vi "Teleop.vi"(10 "Match Info":T1={"Autonomous Elapsed Seconds"=0.0, "TeleOp Elapsed Seconds"=0.0, "Disabled Elapsed Seconds"=0.0, "Visited Autonomous"=FALSE, "Visited TeleOp"=FALSE, "Visited Disabled"=FALSE, "Autonomous Settings"={"Autonomous Style"=enum."Independent", "VI Refnum"=refnum}}, 11 "Call Context":T2) -> ()   [LabVIEW 2013]
doc: "This VI is called for each TeleOp packet received from the DS where the robot is not disabled. It is often used to read from the joysticks and update I/O or to update setpoints for timed control loops. It should complete and return within 20 milliseconds or it may miss DS packets."
uses:
  <vilib>/Rock Robotics/WPI/DriverStation/WPI_DriverStationDerivedRobotMode.ctl
  <vilib>/Rock Robotics/WPI/DriverStation/WPI_DriverStationMatch Info.ctl
  <vilib>/Rock Robotics/WPI/Solenoid/WPI_SolenoidValue.ctl
  <vilib>/Rock Robotics/WPI/Relay/WPI_RelayValue.ctl
  Robot Global Data.vi
  <vilib>/Rock Robotics/WPI/Joystick/WPI_JoystickGetSetRefNum.vi
  <vilib>/Rock Robotics/WPI/Solenoid/WPI_SolenoidSetEnum.vi
panel:
  in  "StatusOfFiringMechanism":enum16{"Retracting", "Extending", "Off", ""}(ring)=enum."Off"
  in  "PID Distance":dbl
  in  "Run PID":bool
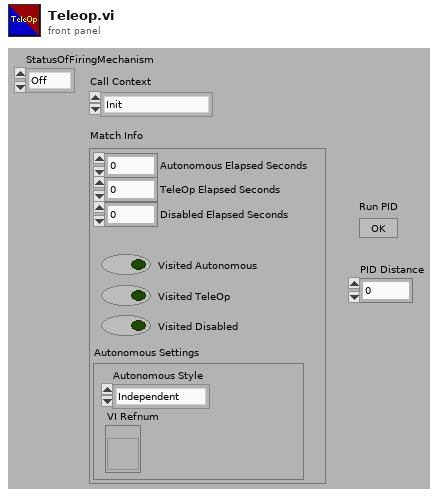
[diagram p1: front panel]
types:
  T1 = typedef "WPI_DriverStationMatch Info.ctl" = cluster{"Autonomous Elapsed Seconds":dbl, "TeleOp Elapsed Seconds":dbl, "Disabled Elapsed Seconds":dbl, "Visited Autonomous":bool, "Visited TeleOp":bool, "Visited Disabled":bool, "Autonomous Settings":cluster{"Autonomous Style":enum16{"Iterative", "Independent"}, "VI Refnum":refnum<vi>}}
  T2 = typedef "WPI_DriverStationDerivedRobotMode.ctl" = enum16{"Init", "Execute", "Stop"}
  T3 = typedef "WPI_RelayDevRef.ctl" = cluster{"DevStatus":errorcluster, "Relay Channel":T4, "Digital Module":T5, "Relay Direction":T6}
  T4 = typedef "FPGA_DIORelayChannel.ctl" = enum8{"Relay 1", "Relay 2", "Relay 3", "Relay 4", "Relay 5", "Relay 6", "Relay 7", "Relay 8", "Invalid"}
  T5 = typedef "FPGA_TypedefDigitalModule.ctl" = enum16{"Digital Module 1", "Digital Module 2"}
  T6 = typedef "WPI_RelayDirection.ctl" = enum16{"Both directions", "Forward only", "Reverse only"}
  T7 = typedef "WPI_SolenoidDevRef.ctl" = cluster{"DevStatus":errorcluster, "Solenoid Module":T8, "Forward Solenoid Channel":T9, "Reverse Solenoid Channel":T9}
  T8 = typedef "FPGA_TypedefSolenoidModule.ctl" = enum16{"Solenoid Module 1", "Solenoid Module 2"}
  T9 = typedef "WPI_SolenoidChannel.ctl" = enum8{"Solenoid 1", "Solenoid 2", "Solenoid 3", "Solenoid 4", "Solenoid 5", "Solenoid 6", "Solenoid 7", "Solenoid 8", "Invalid"}
  T10 = typedef "WPI_RelayValue.ctl" = enum16{"Off", "On", "Forward", "Reverse"}
  T11 = typedef "WPI_SolenoidValue.ctl" = enum16{"Off", "On", "Forward", "Reverse"}
  T12 = typedef "WPI_MotorControlDeviceRef.ctl" = cluster{"DeviceStatus":errorcluster, "Type":enum16{"PWM", "CAN"}, "PWM":cluster{"Digital Module":T5, "PWM Channel":T13, "DeadBand":T14}, "CAN":cluster{"Device Number":u8, "Control Mode":T15, "Semaphore":T16, "Max Vout":dbl}, "Invert":bool, "TransformRef":T17, "InvTransformRef":T17}
  T13 = typedef "FPGA_DIOPWMChannel.ctl" = enum8{"PWM 1", "PWM 2", "PWM 3", "PWM 4", "PWM 5", "PWM 6", "PWM 7", "PWM 8", "PWM 9", "PWM 10", "Invalid"}
  T14 = typedef "WPI_PWMDeadband.ctl" = cluster{"Name":string, "maxPositivePwm":i32, "minPositivePwm":i32, "centerPwm":i32, "maxNegativePwm":i32, "minNegativePwm":i32, "angularRange":u16}
  T15 = typedef "WPI_CANJaguar_ControlMode.ctl" = enum8{"Percent VBus", "Current", "Speed", "Position", "Voltage"}
  T16 = typedef "Semaphore RefNum" = refnum<k1>
  T17 = typedef "WPI_PWMTransform_ConPane.ctl" = refnum<vi>
  T18 = typedef "WPI_RobotDriveDevRef.ctl" = cluster{"DevStatus":errorcluster, "Motors[]":T12[], "Square Inputs":bool, "Max Output":dbl, "Isochronous":bool}
  T19 = typedef "WPI_JoystickDevRef.ctl" = cluster{"Device":T20}
  T20 = typedef "WPI_JoystickDeviceEnum.ctl" = enum16{"USB 1", "USB 2", "USB 3", "USB 4", "Kinect 1", "Kinect 2"}
  T21 = typedef "WPI_JoystickButtonState.ctl" = cluster{"Button 1":bool, "Button 2":bool, "Button 3":bool, "Button 4":bool, "Button 5":bool, "Button 6":bool, "Button 7":bool, "Button 8":bool, "Button 9":bool, "Button 10":bool, "Button 11":bool, "Button 12":bool}
  T22 = cluster{"axis 1 (x)":dbl, "axis 2 (y)":dbl, "axis 3 (throttle)":dbl, "axis 4":dbl, "axis 5":dbl, "axis 6":dbl}
  T23 = typedef "WPI_DigitalInputDevRef.ctl" = cluster{"DevStatus":errorcluster, "DIO Channel":T24, "Digital Module":T5}
  T24 = typedef "FPGA_DIOChannel.ctl" = enum8{"DIO 1", "DIO 2", "DIO 3", "DIO 4", "DIO 5", "DIO 6", "DIO 7", "DIO 8", "DIO 9", "DIO 10", "DIO 11", "DIO 12", "DIO 13", "DIO 14", "Invalid"}
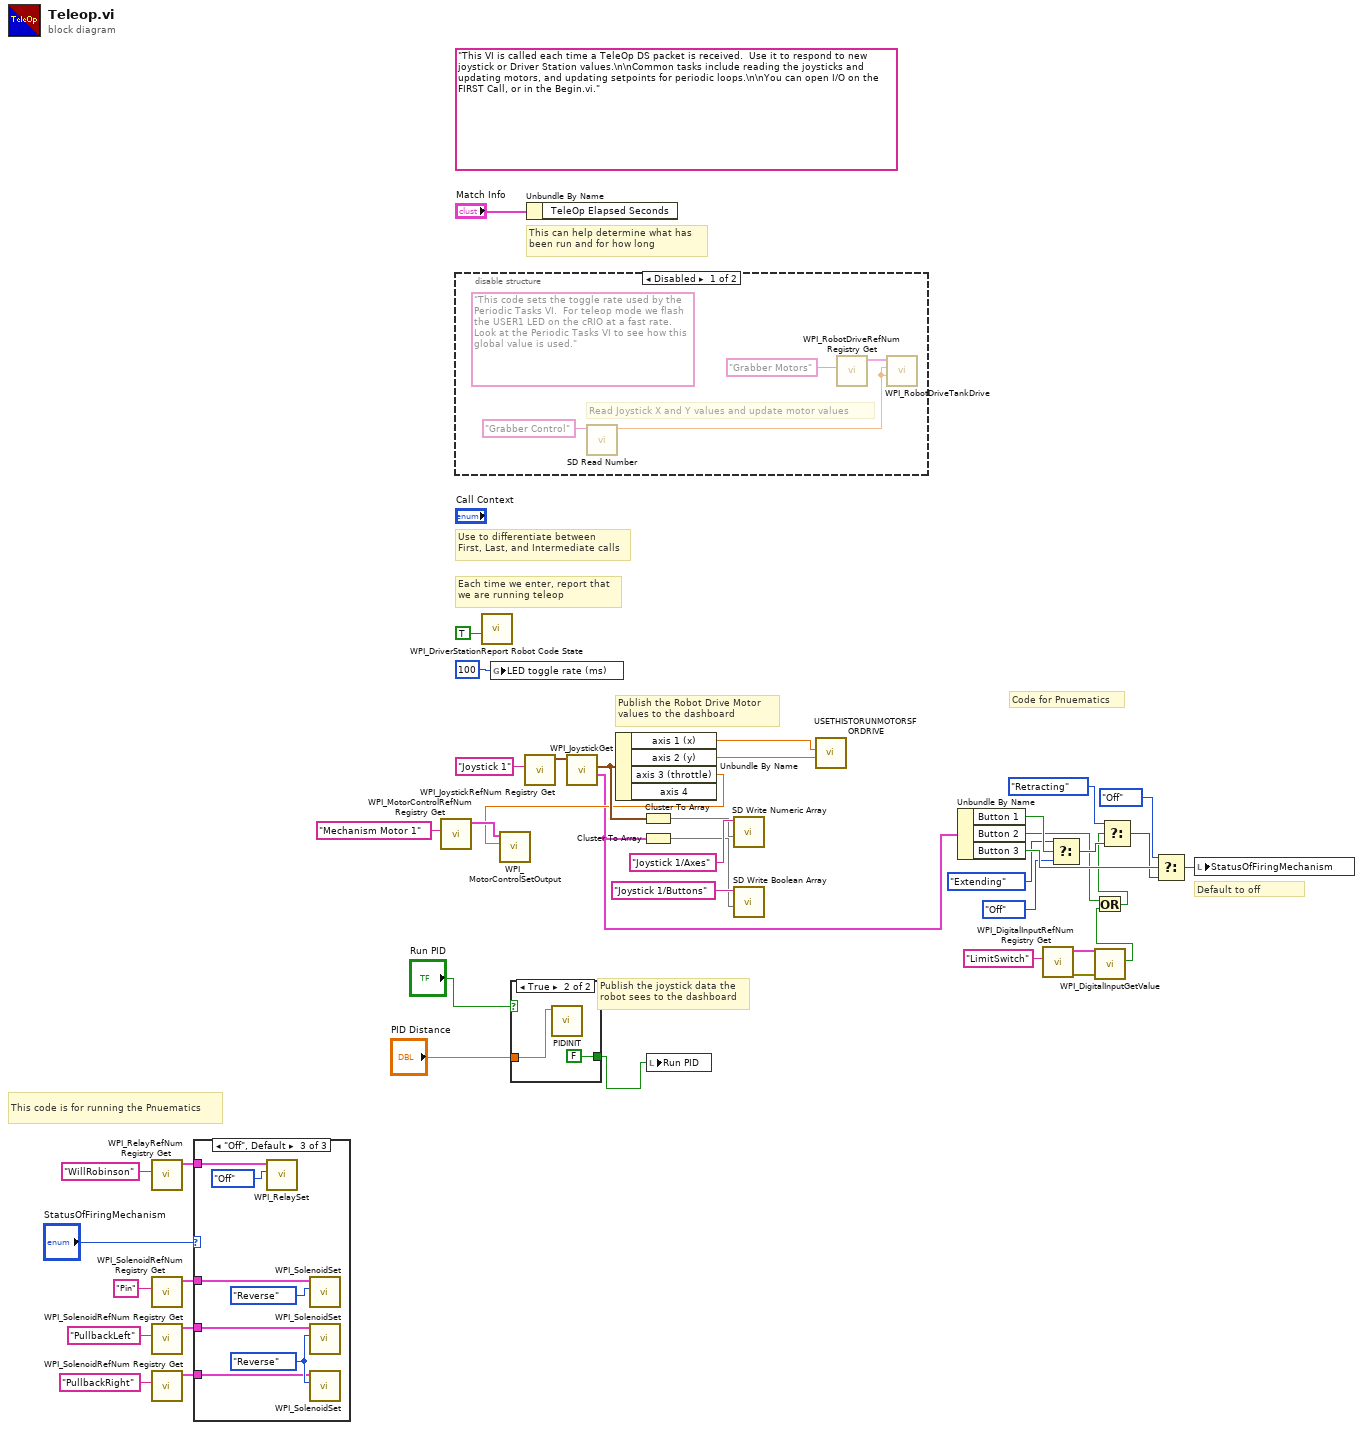
[diagram p0: block diagram]
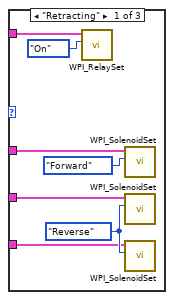
[diagram p2: hidden frame]
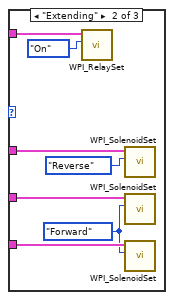
[diagram p3: hidden frame]
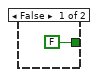
[diagram p4: hidden frame]
diagram:
  (unwired) "This VI is called each time a TeleOp DS packet is received.  Use it to respond to new joystick or Driver Station values.\n\nCommon tasks include reading the joysticks and updating motors, and updating setpoints for periodic loops.\n\nYou can open I/O on the FIRST Call, or in the Begin.vi."
  # "Code for Pnuematics"
  # "Default to off"
  # "This code is for running the Pnuematics"
  # "Publish the Robot Drive Motor\nvalues to the dashboard"
  # "Publish the joystick data the\nrobot sees to the dashboard"
  # "Each time we enter, report that\nwe are running teleop"
  # "Use to differentiate between\nFirst, Last, and Intermediate calls"
  # "This can help determine what has\nbeen run and for how long"
  n1 = call <vilib>:"WPI_RelayRefNum Registry Get.vi"("refnum name"="WillRobinson") -> ("RelayDevRef"=w7:T3)  [unwired: 9 in, 1 out]
  n2 = call <vilib>:"WPI_SolenoidRefNum Registry Get.vi"("refnum name"="Pin") -> ("SolenoidDevRef"=w8:T7)  [unwired: 9 in, 1 out]
  n3 = call <vilib>:"WPI_SolenoidRefNum Registry Get.vi"("refnum name"="PullbackLeft") -> ("SolenoidDevRef"=w21:T7)  [unwired: 9 in, 1 out]
  n4 = call <vilib>:"WPI_SolenoidRefNum Registry Get.vi"("refnum name"="PullbackRight") -> ("SolenoidDevRef"=w20:T7)  [unwired: 9 in, 1 out]
  n5 = case shown="\"Off\", Default" "StatusOfFiringMechanism" {
    tunnel: w21 -> [w46 w57 w60]
    tunnel: w20 -> [w47 w56 w61]
    tunnel: w8 -> [w45 w53 w59]
    tunnel: w7 -> [w44 w52 w58]
    frame "Retracting" {
      w48 = WPI_SolenoidValue."Reverse" ("Value")
      n6 = call <vilib>:"WPI_RelaySet.vi"("RelayValue"=WPI_RelayValue."On", "RelayDevRef"=w44) -> ()  [unwired: 8 in, 2 out]
      n7 = call-poly <vilib>:"WPI_SolenoidSet.vi"("Value"=WPI_SolenoidValue."Forward", "SolenoidDevRef"=w45) -> ()  [unwired: 8 in, 2 out]
      n8 = call-poly <vilib>:"WPI_SolenoidSet.vi"("Value"=w48, "SolenoidDevRef"=w46) -> ()  [unwired: 8 in, 2 out]
      n9 = call-poly <vilib>:"WPI_SolenoidSet.vi"("Value"=w48, "SolenoidDevRef"=w47) -> ()  [unwired: 8 in, 2 out]
    }
    frame "Extending" {
      w55 = WPI_SolenoidValue."Forward" ("Value")
      n10 = call <vilib>:"WPI_RelaySet.vi"("RelayValue"=WPI_RelayValue."On", "RelayDevRef"=w52) -> ()  [unwired: 8 in, 2 out]
      n11 = call-poly <vilib>:"WPI_SolenoidSet.vi"("Value"=WPI_SolenoidValue."Reverse", "SolenoidDevRef"=w53) -> ()  [unwired: 8 in, 2 out]
      n12 = call-poly <vilib>:"WPI_SolenoidSet.vi"("Value"=w55, "SolenoidDevRef"=w57) -> ()  [unwired: 8 in, 2 out]
      n13 = call-poly <vilib>:"WPI_SolenoidSet.vi"("Value"=w55, "SolenoidDevRef"=w56) -> ()  [unwired: 8 in, 2 out]
    }
    frame "Off", Default {
      w62 = WPI_SolenoidValue."Reverse" ("Value")
      n14 = call <vilib>:"WPI_RelaySet.vi"("RelayValue"=WPI_RelayValue."Off", "RelayDevRef"=w58) -> ()  [unwired: 8 in, 2 out]
      n15 = call-poly <vilib>:"WPI_SolenoidSet.vi"("Value"=WPI_SolenoidValue."Reverse", "SolenoidDevRef"=w59) -> ()  [unwired: 8 in, 2 out]
      n16 = call-poly <vilib>:"WPI_SolenoidSet.vi"("Value"=w62, "SolenoidDevRef"=w60) -> ()  [unwired: 8 in, 2 out]
      n17 = call-poly <vilib>:"WPI_SolenoidSet.vi"("Value"=w62, "SolenoidDevRef"=w61) -> ()  [unwired: 8 in, 2 out]
    }
  }
  n18 = call <vilib>:"WPI_MotorControlRefNum Registry Get.vi"("refnum name"="Mechanism Motor 1") -> ("MotorControlDevRef"=w30:T12)  [unwired: 9 in, 1 out]
  n19 = disable-structure shown="Disabled" {
    frame Disabled {
      (unwired) "This code sets the toggle rate used by the Periodic Tasks VI.  For teleop mode we flash the USER1 LED on the cRIO at a fast rate.  Look at the Periodic Tasks VI to see how this global value is used."
      # "Read Joystick X and Y values and update motor values"
      n20 = call <vilib>:"SD Read Number.vi"("Name"="Grabber Control") -> ("Numeric"=w65:dbl)  [unwired: 8 in, 2 out]
      n21 = call <vilib>:"WPI_RobotDriveRefNum Registry Get.vi"("refnum name"="Grabber Motors") -> ("RobotDriveDevRef"=w66:T18)  [unwired: 9 in, 1 out]
      n22 = call <vilib>:"WPI_RobotDriveTankDrive.vi"("Right axis value"=w65, "Left axis value"=w65, "RobotDriveDevRef"=w66) -> ()  [unwired: 6 in, 3 out]
    }
    frame Enabled {
    }
  }
  n23 = call <vilib>:"WPI_DriverStationReport Robot Code State.vi"("TeleOp"=TRUE ("Autonomous")) -> ()  [unwired: 10 in, 1 out]
  n24 = global write "Robot Global Data.vi" "LED toggle rate (ms)"(u32 100 ("LED ms toggle rate")) -> ()
  n25 = case shown="True" "Run PID" {
    tunnel: [FALSE ("Run PID") FALSE ("Run PID")] -> w28
    tunnel: "PID Distance" -> [_ w70]
    frame False {
    }
    frame True {
      n26 = call "PIDINIT.vi"("setpoint"=w70) -> ()  [unwired: 11 in]
    }
  }
  n27 = call <vilib>:"WPI_JoystickRefNum Registry Get.vi"("refnum name"="Joystick 1") -> ("JoystickDevRef"=w35:T19)  [unwired: 1 in, 9 out]
  n28 = Unbundle By Name("Match Info") -> ()  [unwired: 1 out]
  n29 = call <vilib>:"WPI_JoystickGet.vi"("JoystickDevRef"=w35) -> ("Buttons"=w18:T21, "Axes"=w38:T22)  [unwired: 1 in, 4 out]
  n30 = Unbundle By Name(w38) -> ("axis 1 (x)"=w33:dbl, "axis 2 (y)"=w32:dbl, "axis 3 (throttle)"=w29:dbl)  [unwired: 1 out]
  n31 = call <vilib>:"WPI_MotorControlSetOutput.vi"("Output"=w29, "MotorControlDevRef"=w30) -> ()  [unwired: 7 in, 3 out]
  n32 = Cluster To Array(cluster=w38) -> (array=w39:dbl[])
  n33 = Cluster To Array(cluster=w18) -> (array=w36:bool[])
  n34 = local write "Run PID"(w28) -> ()
  n35 = call <vilib>:"SD Write Numeric Array.vi"("Numeric Array"=w39, "Name"="Joystick 1/Axes") -> ()  [unwired: 8 in, 2 out]
  n36 = call <vilib>:"SD Write Boolean Array.vi"("Boolean Array"=w36, "Name"="Joystick 1/Buttons") -> ()  [unwired: 8 in, 2 out]
  n37 = call "USETHISTORUNMOTORSFORDRIVE.vi"("Y axis value"=w32, "X axis value"=w33) -> ()  [unwired: 10 in]
  n38 = Unbundle By Name(w18) -> ("Button 1"=w16:bool, "Button 2"=w2:bool, "Button 3"=w17:bool)
  n39 = call <vilib>:"WPI_DigitalInputRefNum Registry Get.vi"("refnum name"="LimitSwitch") -> ("error out"=w5:errorcluster, "DigitalInputDevRef"=w4:T23)  [unwired: 9 in]
  n40 = Select(t=enum16{"Retracting", "Extending", "Off", ""}."Extending" ("StatusOfFiringMechanism"), s=w16, f=enum16{"Retracting", "Extending", "Off", ""}."Off" ("StatusOfFiringMechanism")) -> (s? t:f=w13:enum16{"Retracting", "Extending", "Off", ""})
  n41 = call <vilib>:"WPI_DigitalInputGetValue.vi"("error in (no error)"=w5, "DigitalInputDevRef"=w4) -> ("Value"=w3:bool)  [unwired: 7 in, 2 out]
  n42 = Or(x=w2, y=w3) -> (x .or. y?=w1:bool)
  n43 = Select(t=enum16{"Retracting", "Extending", "Off", ""}."Retracting" ("StatusOfFiringMechanism"), s=w1, f=w13) -> (s? t:f=w14:enum16{"Retracting", "Extending", "Off", ""})
  n44 = Select(t=enum16{"Retracting", "Extending", "Off", ""}."Off" ("StatusOfFiringMechanism"), s=w17, f=w14) -> (s? t:f=w15:enum16{"Retracting", "Extending", "Off", ""})
  n45 = local write "StatusOfFiringMechanism"(w15) -> ()
